vi "Pemula 4.vi"() -> (0 "Boolean 2":bool, 2 "Password 2":string, 3 "Username 2":string)   [LabVIEW 2017]
panel:
  in  "Boolean":bool
  in  "Password":string
  in  "Username":string
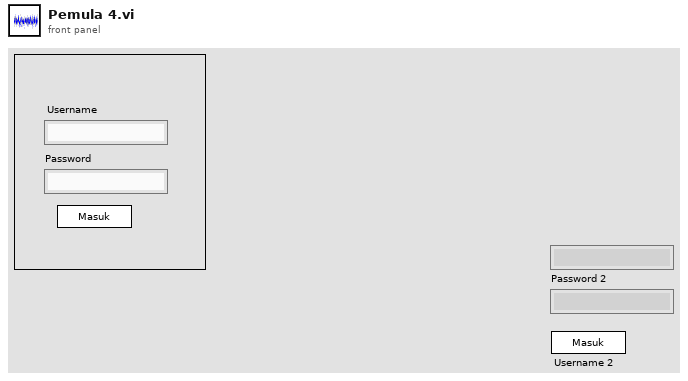
[diagram p1: front panel]
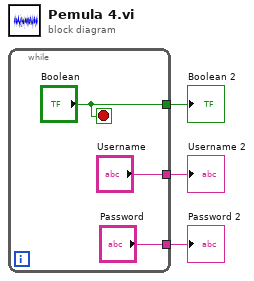
[diagram p0: block diagram]
diagram:
  n1 = while {
    tunnel: ["Boolean"] -> w3
    tunnel: ["Username"] -> w2
    tunnel: ["Password"] -> w1
    stop <- "Boolean" stop-if-true
  }
  "Boolean 2" <- w3
  "Username 2" <- w2
  "Password 2" <- w1
